vi "Configure Waveform (Sinusoid).vi"(0 "VISA resource name":refnum<visa-resource-name>, 1 "Amplitude (0)":dbl, 2 "Offset Level (0)":dbl, 3 "Enable Trigger Output (T: Enable)":bool=TRUE, 5 "Output Channel (0: Channel 1)":i32(ring) items=["Channel 1", "Channel 2"], 7 "Source Mode (1: Voltage)":i32(ring)=1 items=["Current", "Voltage"], 9 "Trigger Output Port (0: External1)":i32(ring) items=["External1", "External2", "External3", "External4", "External5", "External6", "External7", "External8", "External9", "External10", "External11", "External12", "External13", "External14", "Internal1", "Internal2"], 11 "error in (no error)":errorcluster, 12 "Frequency (0.001 Hz)":dbl=0.001, 13 "Phase Marker (0 Degree)":dbl) -> (4 "VISA resource name out":refnum<visa-resource-name>, 15 "error out":errorcluster)   [LabVIEW 2020, in "Agilent B2900 Series.lvlib"]
doc: "Configure current or voltage sinusoid waveform output.\n\n<B>Note:</B>\nThis VI is only supported by Agilent models B2961A, B2962A, B2961B and B2962B."
uses:
  Agilent B2900 Series.lvlib
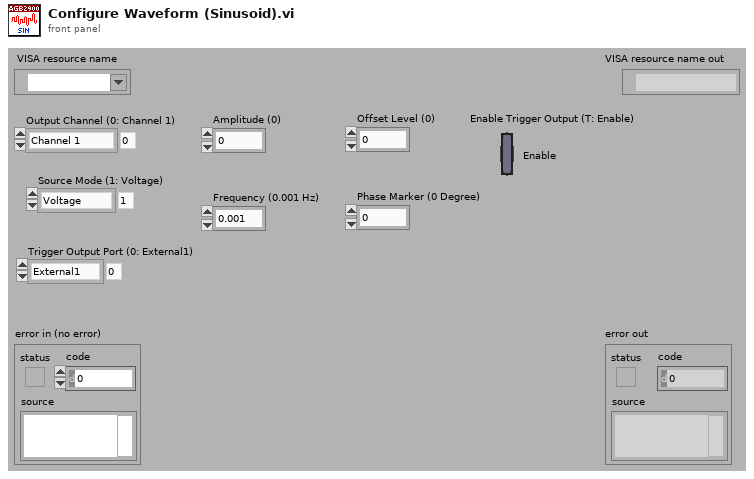
[diagram p1: front panel]
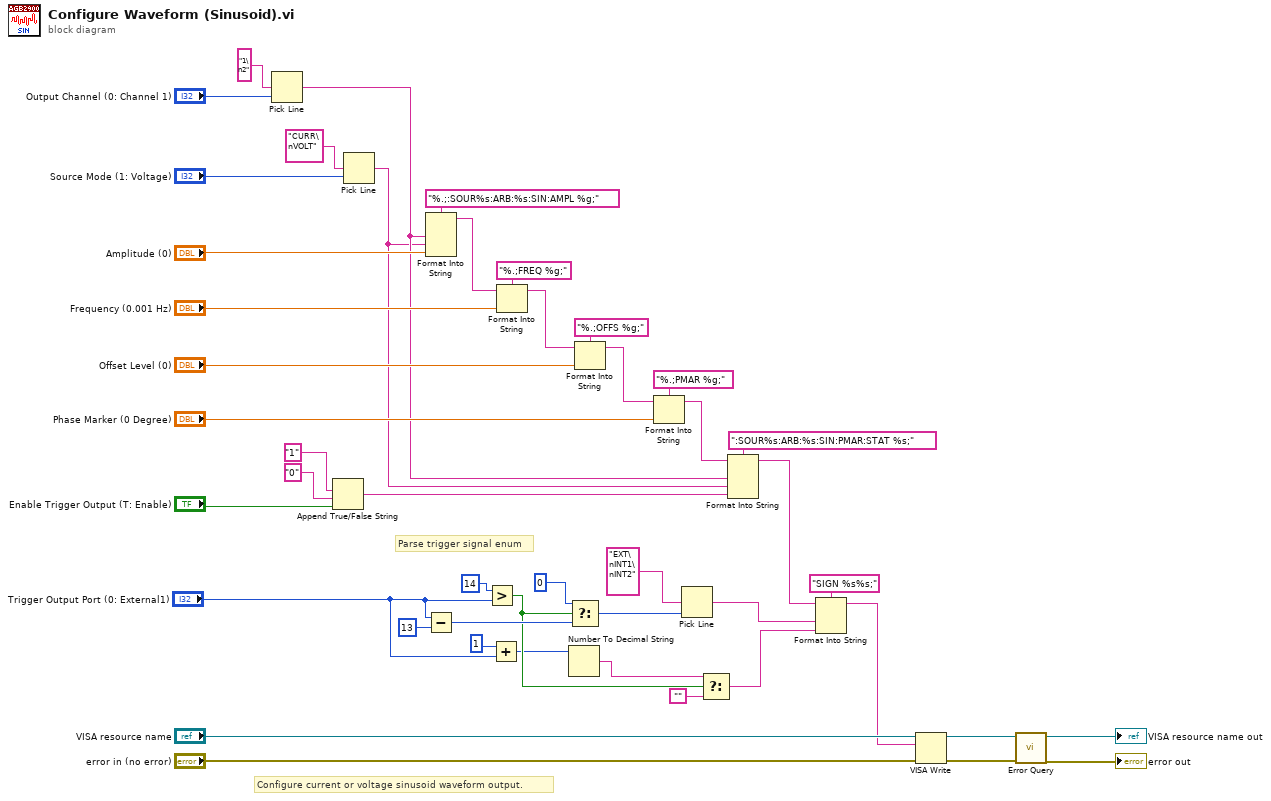
[diagram p0: block diagram]
diagram:
  # "Parse trigger signal enum"
  # "Configure current or voltage sinusoid waveform output."
  n1 = Pick Line(multi-line string="1\n2", line index="Output Channel (0: Channel 1)") -> (output string=w10:string)  [unwired: 1 in]
  n2 = Append True/False String(1:"Enable Trigger Output (T: Enable)", 2:"0", 3:"1") -> (0:w8:string)  [unwired: 1 out]
  n3 = Pick Line(multi-line string="CURR\nVOLT", line index="Source Mode (1: Voltage)") -> (output string=w9:string)  [unwired: 1 in]
  n4 = Format Into String(format string="%.;:SOUR%s:ARB:%s:SIN:AMPL %g;", w10, w9, "Amplitude (0)") -> (resulting string=w24:string)  [unwired: 2 in, 1 out]
  n5 = Subtract(x="Trigger Output Port (0: External1)", y=13) -> (x-y=w17:i32)
  n6 = Greater?(x=14 ("y"), y="Trigger Output Port (0: External1)") -> (0:w14:bool)
  n7 = Add(x=1, y="Trigger Output Port (0: External1)") -> (x+y=w12:i32)
  n8 = Format Into String(format string="%.;FREQ %g;", initial string=w24, "Frequency (0.001 Hz)") -> (resulting string=w23:string)  [unwired: 1 in, 1 out]
  n9 = Number To Decimal String(number=w12) -> (decimal integer string=w20:string)  [unwired: 1 in]
  n10 = Select(t=0, s=w14, f=w17) -> (s? t:f=w19:i32)
  n11 = Format Into String(format string="%.;OFFS %g;", initial string=w23, "Offset Level (0)") -> (resulting string=w7:string)  [unwired: 1 in, 1 out]
  n12 = Format Into String(format string="%.;PMAR %g;", initial string=w7, "Phase Marker (0 Degree)") -> (resulting string=w6:string)  [unwired: 1 in, 1 out]
  n13 = Pick Line(multi-line string="EXT\nINT1\nINT2", line index=w19) -> (output string=w5:string)  [unwired: 1 in]
  n14 = Select(t=w20, s=w14, f="") -> (s? t:f=w4:string)
  n15 = Format Into String(format string=":SOUR%s:ARB:%s:SIN:PMAR:STAT %s;", initial string=w6, w10, w9, w8) -> (resulting string=w3:string)  [unwired: 1 in, 1 out]
  n16 = Format Into String(format string="SIGN %s%s;", initial string=w3, w5, w4) -> (resulting string=w2:string)  [unwired: 1 in, 1 out]
  n17 = VISA Write(VISA resource name="VISA resource name", write buffer=w2, error in (no error)="error in (no error)") -> (VISA resource name out=w31:refnum<visa-resource-name>, error out=w30:errorcluster)  [unwired: 1 out]
  n18 = call "Error Query.vi"("error in (no error)"=w30, "VISA resource name"=w31) -> ("error out"=→"error out":errorcluster, "VISA resource name out"=→"VISA resource name out":refnum<visa-resource-name>)  [unwired: 8 out]
